vi "NML Spectrum Analyzer.vi"(1 "Channel Selector":i16(slide) scale=0.0..7.0, 2 "# of Samples":u32(slide)=5 scale=0.0..8.0) -> (3 "WAVEFORM":dbl[](graph), 4 "POWER SPECTRUM":cluster{ext, dbl, dbl[]}(graph), 5 "SPECTRUM DATA":dbl[](array[numeric])=[7.585612974564393e-07] format="%.4e", 6 "F= 1/(NÆt)":dbl=4.8828125 format="%.4f")   [LabVIEW 2021]
doc: "This VI uses the NML Oscilloscope VI to acquire a waveform then computes its power spectrum.\nScott Hannahs, FBNML,Jan 1992"
panel:
  in  "Gain":dbl(slide) scale=0.0..3.0 scale format="%.2f"
  in  "Filter Type":T1(ring)=enum."Hanning"
  in  "Sample period\n     msec":dbl=0.1 format="%.4f"
  # "Volts"
  # "Time (msec)"
  # "Frequency (Hz)"
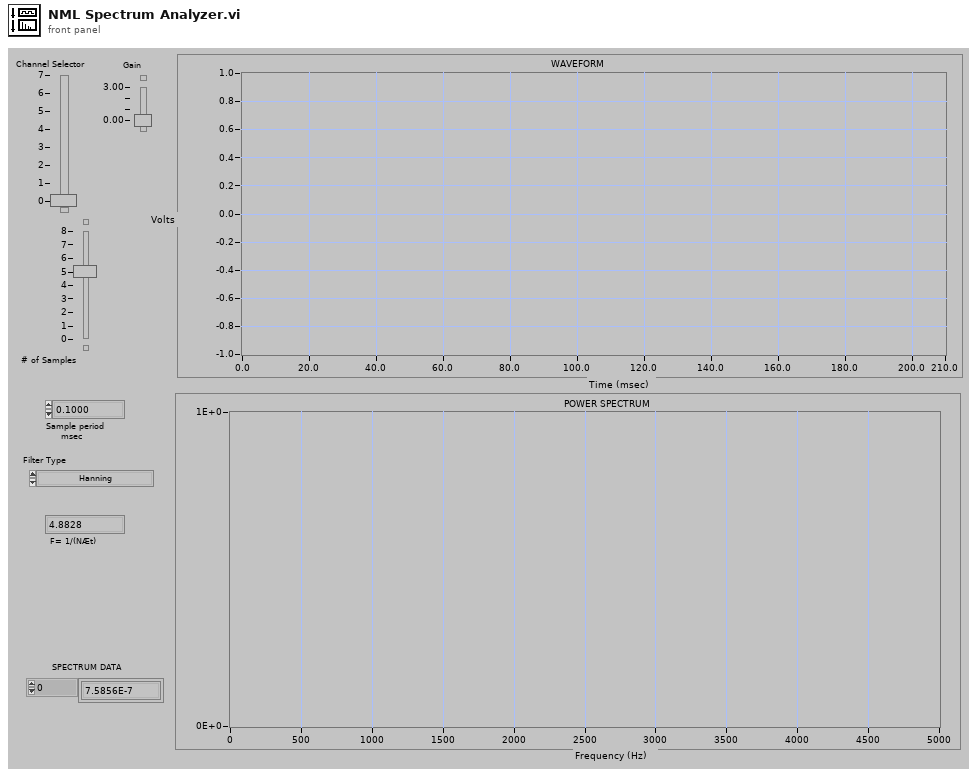
[diagram p1: front panel]
types:
  T1 = enum16{"None", "Hanning", "Hamming", "Kaiser-Bessel", "Flat Top", "Triangle", "Genral Cosine", "Cosine Tapered", "Blackman", "Exact Blackman", "Blackman-Harris"}
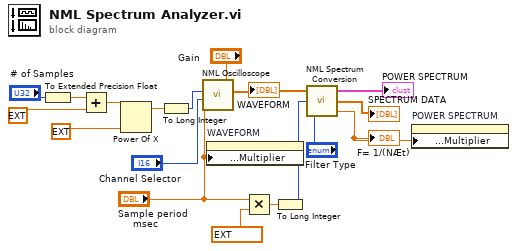
[diagram p0: block diagram]
diagram:
  n1 = To Extended Precision Float(1:"# of Samples") -> (0:w8:ext)
  n2 = Add(x=w8, y=ext 6.0) -> (x+y=w9:ext)
  n3 = Power Of X(1:ext 2.0, 2:w9) -> (0:w13:ext)
  n4 = To Long Integer(number=w13) -> (32bit integer=w6:i32)
  n5 = call "NML Oscilloscope.vi"("Range Max"="Gain", "Time Between\nSamples (msec)"="Sample period\n     msec", "Chan #"="Channel Selector", "Number of Samples"=w6) -> ("WAVEFORM SAMPLES"=w2:dbl[])  [unwired: 4 in, 1 out]
  "WAVEFORM" <- w2
  n6 = property on="WAVEFORM" class="WFGraph (strict)"("X Scale.Offset and Multiplier:Multiplier"="Sample period\n     msec") -> ()  [unwired: 2 in, 2 out]
  n7 = Multiply(x="Sample period\n     msec", y=ext 1000.0) -> (x*y=w5:ext)
  n8 = To Long Integer(number=w5) -> (32bit integer=w3:i32)
  n9 = call "NML Spectrum Conversion.vi"("Filter Type"="Filter Type", "DELTA TIME µSec"=w3, "WAVEFORM DATA"=w2) -> ("FREQUENCY \nRESOLUTION"=w18:dbl, "SPECTRUM DATA"=→"SPECTRUM DATA":dbl[], "SPECTRUM"=→"POWER SPECTRUM":cluster{ext, dbl, dbl[]})
  "F= 1/(NÆt)" <- w18
  n10 = property on="POWER SPECTRUM" class="WFGraph (strict)"("X Scale.Offset and Multiplier:Multiplier"=w18) -> ()  [unwired: 2 in, 2 out]
